vi "Create OPCUA Server Auto.vi"(8 "Error In":errorcluster, 11 "XML config File Path":path=path "D:/work/Project support in lanzhou/OPCUA XML/xml/server config.xml") -> (0 "Error Out":errorcluster, 1 "Parse Errors":string, 2 "server endpoint URL":string, 3 "OPC UA server refnum out":refnum<k21>, 4 "trusted client certfications":path[](array[path]))   [LabVIEW 2013, in "OPCUA XML.lvlib"]
doc: "This example loads test configuration data from an XML file, and checks to see if it is valid against a specific schema. Select whether you want to load the valid or invalid file and run the VI to see the results."
uses:
  OPCUA XML.lvlib
  <vilib>/xml/NI_XML.lvlib
  <vilib>/xml/Close Reference(Node).vi
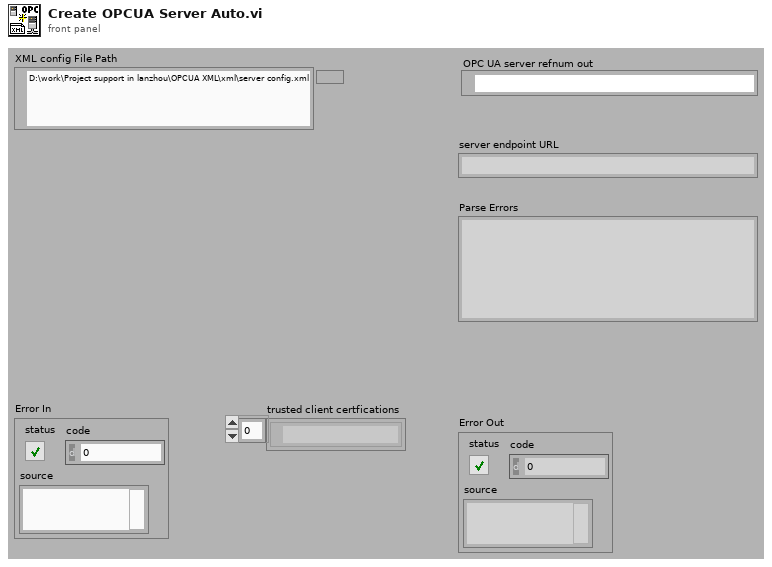
[diagram p1: front panel]
types:
  T1 = typedef "OPCUA XML.lvlib/UA_XML Data.ctl" = cluster{"type":T2, "Data":string}
  T2 = typedef "OPCUA XML.lvlib/UA_RowType.ctl" = enum16{"none", "folder", "item", "property", "folder end", "item end"}
  T3 = typedef "OPCUA XML.lvlib/UA_Server config info.ctl" = cluster{"name":string, "port":string, "policy":string, "serverCertification":string, "trustedClientCertifications":string, "CertificationsFiles":path[]}
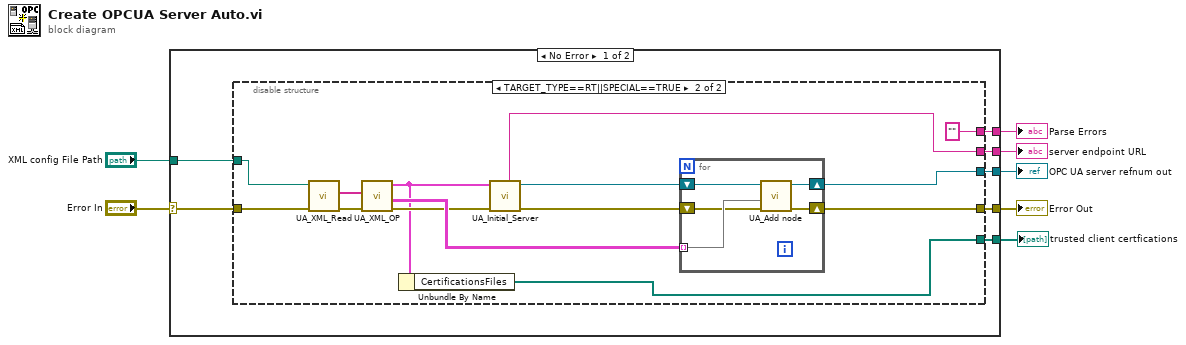
[diagram p0: block diagram]
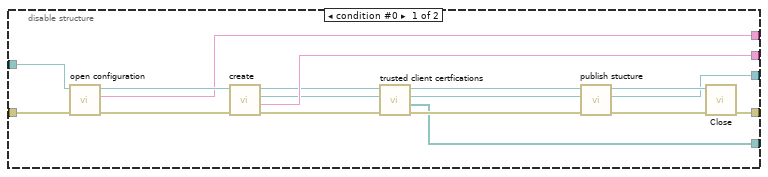
[diagram p2: hidden frame]
diagram:
  n1 = case shown="No Error" "Error In" {
    selector: "Error In" -> [w9 w51]
    tunnel: [w14 w51] -> w7
    tunnel: "XML config File Path" -> [w13 _]
    tunnel: [w12 _] -> w4
    tunnel: [w11 _] -> w3
    tunnel: [w10 _] -> w2
    tunnel: [w8 _] -> w1
    frame No Error {
      n2 = disable-structure shown="TARGET_TYPE==RT||SPECIAL==TRUE" {
        disable-tunnel: [w27 w37] -> w14
        disable-tunnel: w13 -> [w26 w39]
        disable-tunnel: [w25 "" ("Parse Errors")] -> w12
        disable-tunnel: [w24 w35] -> w11
        disable-tunnel: [w23 w38] -> w10
        disable-tunnel: w9 -> [w22 w36]
        disable-tunnel: [w15 w32] -> w8
        frame condition #0 {
          n3 = call "open configuration.vi"("Error In"=w22, "path to XML document"=w26) -> ("Error Out"=w31:errorcluster, "Parse Errors"=w25:string, "DOM document out"=w30:refnum<k20>)  [unwired: 7 in]
          n4 = call "create.vi"("Error In"=w31, "DOM document in"=w30) -> ("Error Out"=w17:errorcluster, "server endpoint URL"=w23:string, "OPC UA server refnum out"=w21:refnum<k21>, "DOM document out"=w19:refnum<k20>)  [unwired: 6 in]
          n5 = call "trusted client certfications.vi"("Error In"=w17, "OPC UA server refnum in"=w21, "DOM document in"=w19) -> ("Error Out"=w16:errorcluster, "trusted client certfications"=w15:path[], "OPC UA server refnum out"=w20:refnum<k21>, "DOM document out"=w18:refnum<k20>)  [unwired: 5 in]
          n6 = call "publish stucture.vi"("Error In"=w16, "OPC UA server refnum in"=w20, "DOM document in"=w18) -> ("Error Out"=w29:errorcluster, "OPC UA server refnum out"=w24:refnum<k21>, "DOM document out"=w28:refnum<k20>)  [unwired: 6 in]
          n7 = call-poly <vilib>:"Close.vi"("error in (no error)"=w29, "node"=w28) -> ("error out"=w27:errorcluster)  [unwired: 7 out]
        }
        frame condition #1 (active) {
          n8 = call "UA_XML_Read.vi"("error in (no error)"=w36, "XML File Path"=w39) -> ("error out"=w41:errorcluster, "xml Data"=w40:string[])  [unwired: 7 in, 1 out]
          n9 = call "UA_XML_OP.vi"("error in (no error)"=w41, "xml Raw Data"=w40) -> ("error out"=w42:errorcluster, "XML Data Out"=w43:T1[][], "Server config info"=w33:T3)  [unwired: 7 in]
          n10 = Unbundle By Name(w33) -> ("CertificationsFiles"=w32:path[])
          n11 = call "UA_Initial_Server.vi"("error in (no error)"=w42, "Server config infor"=w33) -> ("error out"=w45:errorcluster, "OPC UA server refnum out"=w44:refnum<k21>, "server endpoint URL"=w38:string)  [unwired: 7 in]
          n12 = for {
            tunnel: w43 -> [w49] mode=indexing
            shift-right: [w47] -> w37
            shift-left: w45 -> [w48]
            shift-right: [w46] -> w35
            shift-left: w44 -> [w50]
            n13 = call "UA_Add node.vi"("error in (no error)"=w48, "XML Folder"=w49, "OPC UA server refnum in"=w50) -> ("error out"=w47:errorcluster, "OPC UA server refnum out"=w46:refnum<k21>)  [unwired: 7 in]
          }
        }
      }
    }
    frame Error {
    }
  }
  "Error Out" <- w7
  "Parse Errors" <- w4
  "server endpoint URL" <- w2
  "OPC UA server refnum out" <- w3
  "trusted client certfications" <- w1
